vi "MaxMinValues.vi"(2 "BeforeMin":dbl, 3 "Numeric":dbl, 4 "BeforeMax":dbl) -> (0 "Min":dbl, 1 "Max":dbl)   [LabVIEW 2018]
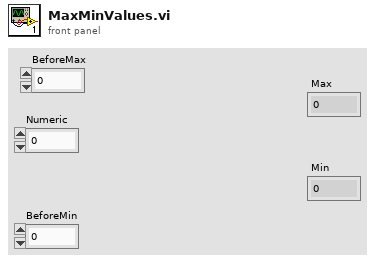
[diagram p1: front panel]
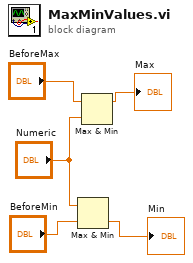
[diagram p0: block diagram]
diagram:
  n1 = Max & Min(x="Numeric", y="BeforeMin") -> (min(x,y)=→"Min":dbl)  [unwired: 1 out]
  n2 = Max & Min(x="BeforeMax", y="Numeric") -> (max(x,y)=→"Max":dbl)  [unwired: 1 out]
